vi "test_PhotonCamera_All.vi"(8 "error in (no error)":errorcluster) -> (0 "error out":errorcluster, 3 "Test Passed":bool)   [LabVIEW 2019]
panel:
  out "Empty Test":bool
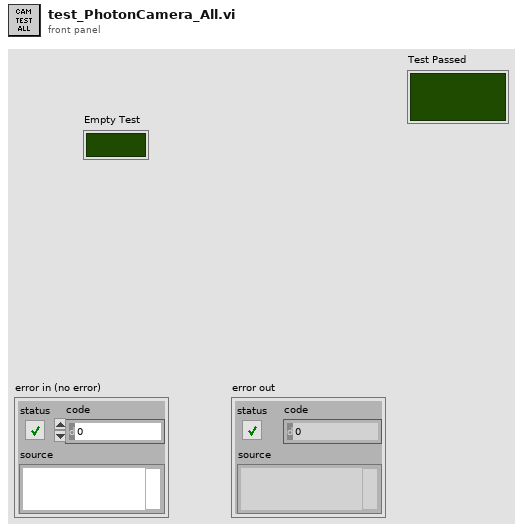
[diagram p1: front panel]
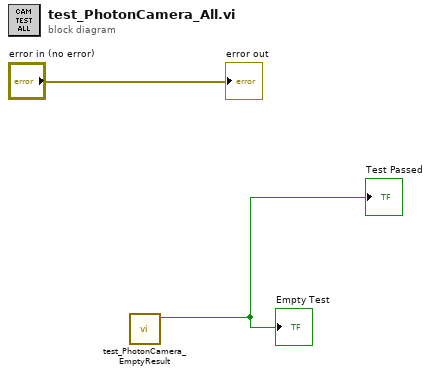
[diagram p0: block diagram]
diagram:
  n1 = call "test_PhotonCamera_EmptyResult.vi"() -> ("Test Passed"=→"Test Passed" →"Empty Test":bool)  [unwired: 10 in, 1 out]
  "error out" <- "error in (no error)"
